vi "read accel data.vi"(8 "error in (no error)":errorcluster, 11 "data":T1) -> (0 "error out":errorcluster, 2 "function return":i32, 3 "data out":T1)   [LabVIEW 2014, in "libroboticscape.lvlib"]
doc: "int read_accel_data(imu_data_t *data);"
uses:
  libroboticscape.lvlib
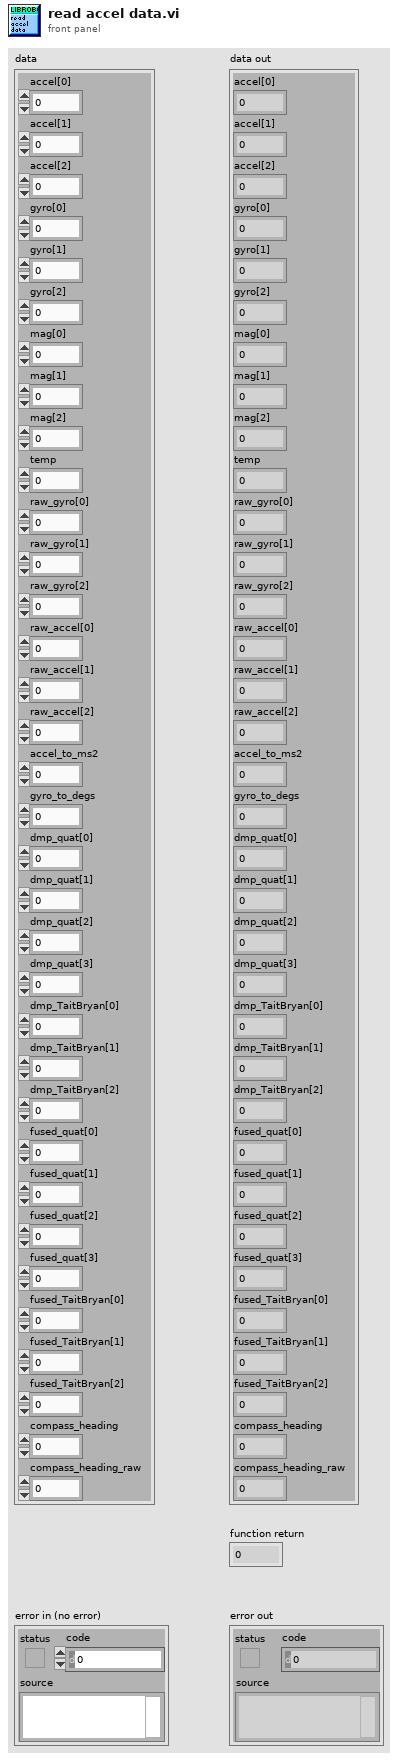
[diagram p1: front panel]
types:
  T1 = cluster{"accel[0]":sgl, "accel[1]":sgl, "accel[2]":sgl, "gyro[0]":sgl, "gyro[1]":sgl, "gyro[2]":sgl, "mag[0]":sgl, "mag[1]":sgl, "mag[2]":sgl, "temp":sgl, "raw_gyro[0]":i16, "raw_gyro[1]":i16, "raw_gyro[2]":i16, "raw_accel[0]":i16, "raw_accel[1]":i16, "raw_accel[2]":i16, "accel_to_ms2":sgl, "gyro_to_degs":sgl, "dmp_quat[0]":sgl, "dmp_quat[1]":sgl, "dmp_quat[2]":sgl, "dmp_quat[3]":sgl, "dmp_TaitBryan[0]":sgl, "dmp_TaitBryan[1]":sgl, "dmp_TaitBryan[2]":sgl, "fused_quat[0]":sgl, "fused_quat[1]":sgl, "fused_quat[2]":sgl, "fused_quat[3]":sgl, "fused_TaitBryan[0]":sgl, "fused_TaitBryan[1]":sgl, "fused_TaitBryan[2]":sgl, "compass_heading":sgl, "compass_heading_raw":sgl}
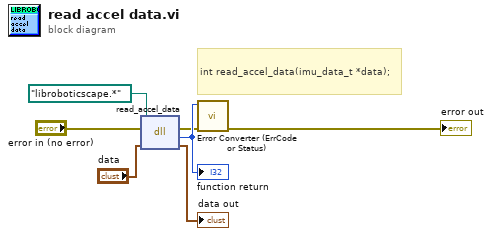
[diagram p0: block diagram]
diagram:
  # "int read_accel_data(imu_data_t *data);"
  n1 = dll-call lib="C:/Users/ktalke/Documents/Robotics-Cape-Master-Jessie/Libroboticscape-Master-Jessie/libroboticscape.so" fn="read_accel_data"(path in=path "libroboticscape.*", error in="error in (no error)", "data"="data") -> (error out=w3:errorcluster, "return type"=w7:i32, "data"=→"data out":T1)  [unwired: 1 in, 1 out]
  "function return" <- w7
  n2 = call "Error Converter (ErrCode or Status).vi"("error in (no error)"=w3, "error code"=w7) -> ("error out"=→"error out":errorcluster)  [unwired: 9 in]
